vi "AWSEXE.vi"(8 "error in (no error)":errorcluster, 11 "DUT":string) -> (0 "error in (out)":errorcluster, 2 "Result":string)   [LabVIEW 2024, in "AWSEXE.lvlib"]
doc: "This template is for the Queued Message Handler design pattern.\n\nThe Event Handling Loop generates messages based on user interface actions.\n\nThe Message Handling Loop processes messages generated by the Event Handling Loop, or by other messages. The messages are string values, so new messages can be added easily to the Message Cases case structure in the Message Handling Loop. Each message cluster can also provide an optional value for Message Data, which is a variant that can be converted to whatever message-specific data is required."
uses:
  AWSEXE.lvlib
  support/Neoway_ctrl.ctl
  controls/Neoway UI Data.ctl
  PrivateControls/FGV_Queue_Control.ctl
  <vilib>/Utility/error.llb/Error Cluster From Error Code.vi
  <vilib>/ErrorRing/Error Ring.xnode
  support/Message Queue/Neoway Message Queue.lvlib
  support/User Event - Stop/72-13360 User Event - Stop.lvlib
  Launcher/Launcher_DTU.lvlib
panel:
  in  "Neoway Flashing":T1
  in  "Config":string
  in  "Read_Res":bool
  in  "Read_Current":bool
  in  "Read_File":bool
  in  "Flash":bool
  out "queue name 2":string
  out "queue name":string
  out "Display <Replace Me>":string
  in  "Output":bool
  in  "Init_Neoway":bool
  in  "Exit":bool
  # "These controls have associated \"Value Changed\" events configured in the Event Structure on the diagram.\n\nReplace them (and reconfigure the Event Structure) with the controls you need for your application."
  # "This template is for the Queued Message Handler design pattern.\n\nSee the block diagram for more information on how to use this template."
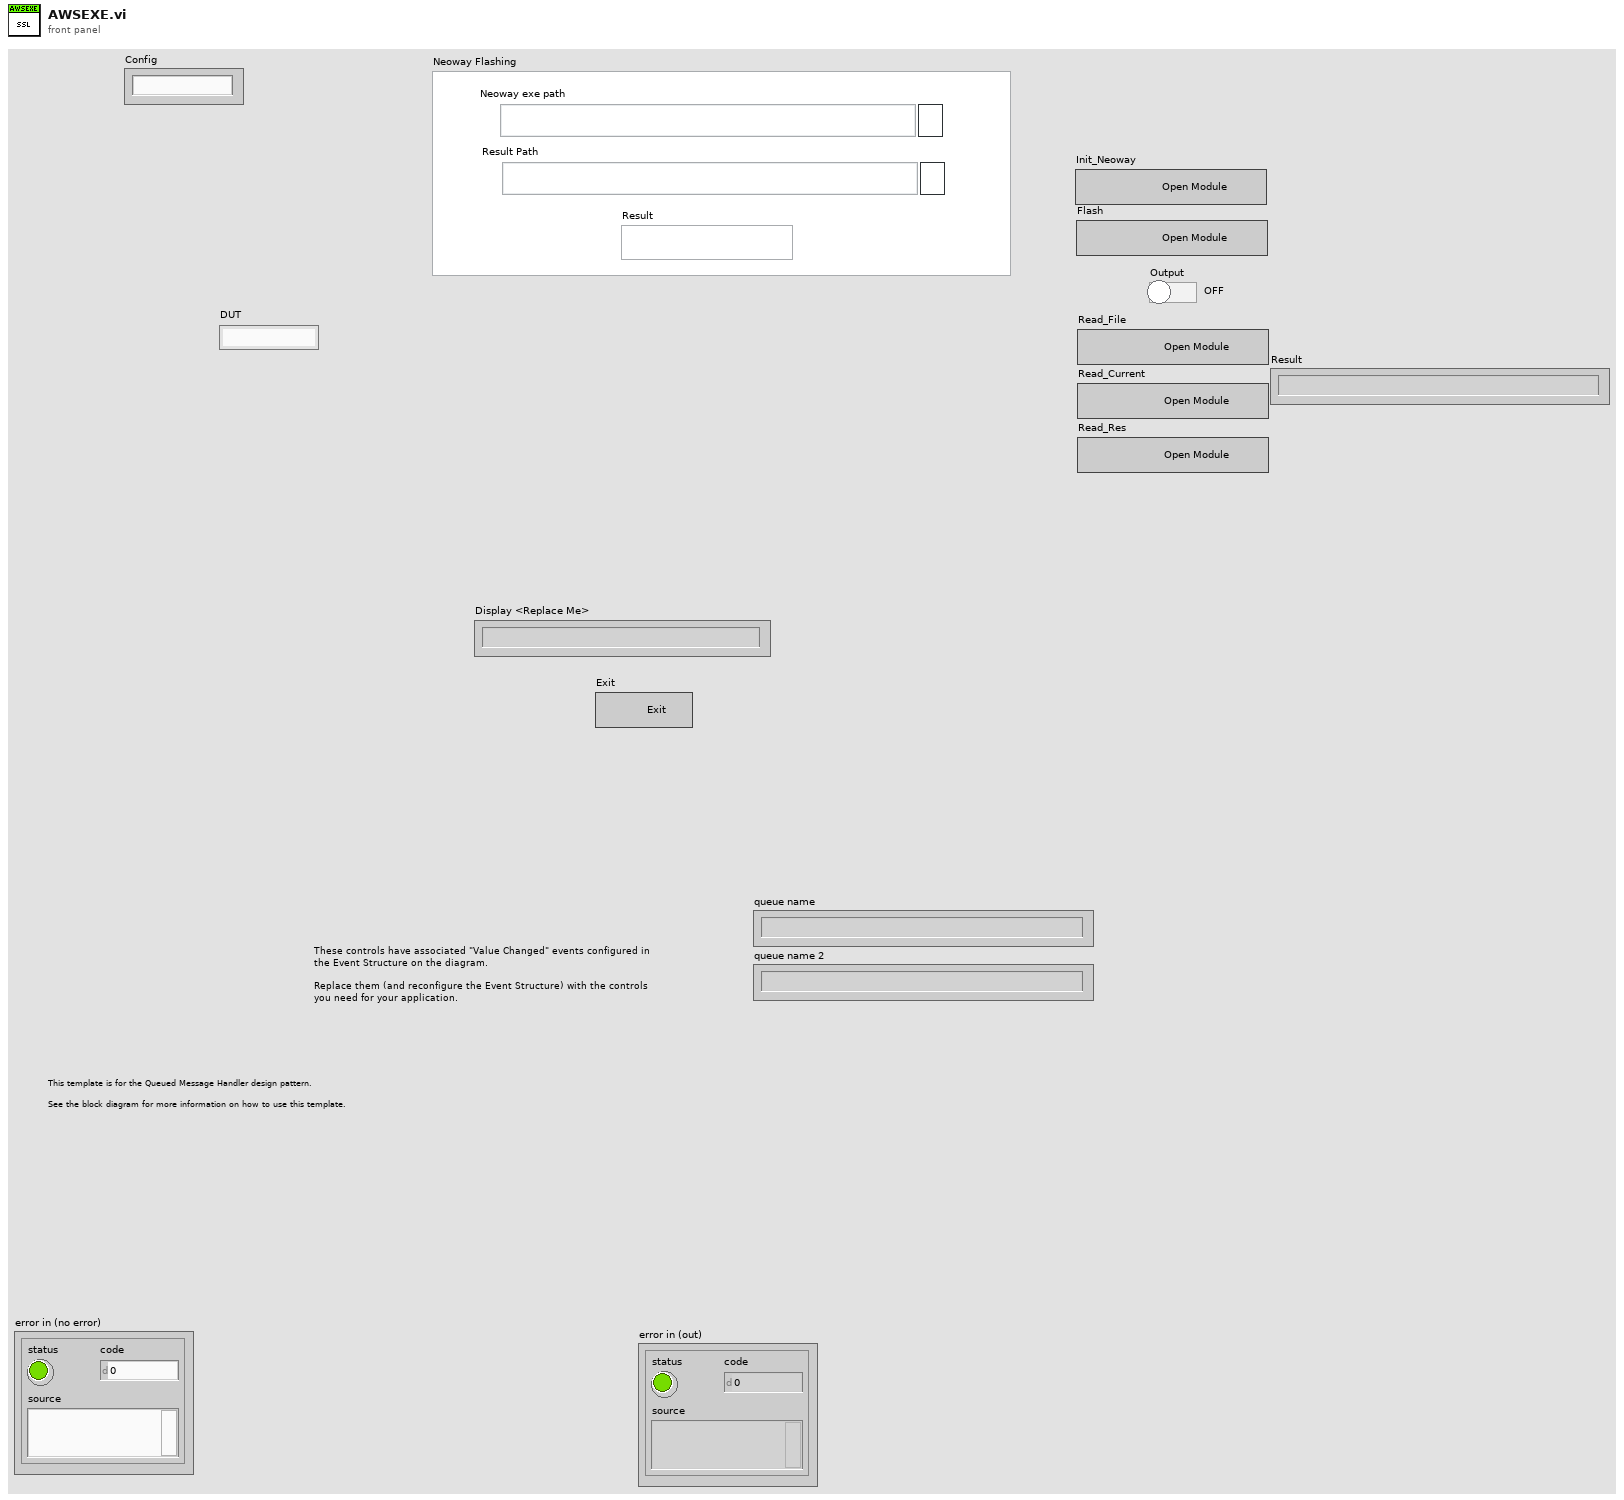
[diagram p1: front panel]
types:
  T1 = typedef "AWSEXE.lvlib/Neoway_ctrl.ctl" = cluster{"Neoway exe path":path, "Result Path":path, "Result":string}
  T2 = typedef "AWSEXE.lvlib/Neoway UI Data.ctl" = cluster{"DUT":string, "Neoway_Q":refnum<queue>, "notifier out":refnum<notifier>, "Config":string, "Neoway Flashing":T1, "Bat file path":path, "Exe path":string, "Flash path":string, "Result":string, "Timer":u32}
  T3 = typedef "AWSEXE.lvlib/FGV_Queue_Control.ctl" = enum16{"Release", "Get", "Set"}
  T4 = typedef "AWSEXE.lvlib/Neoway Message Queue.lvlib/All Message Queues.ctl" = cluster{"UI":refnum<queue>, "QSM":refnum<queue>}
  T5 = cluster{"Message":string, "Message Data":variant}
  T6 = enum16{"Read", "Write", "All_sections", "All_values", "Remove key&section"}
  T7 = enum16{"open", "replace", "create", "open or create", "replace or create", "replace or create with confirmation"}
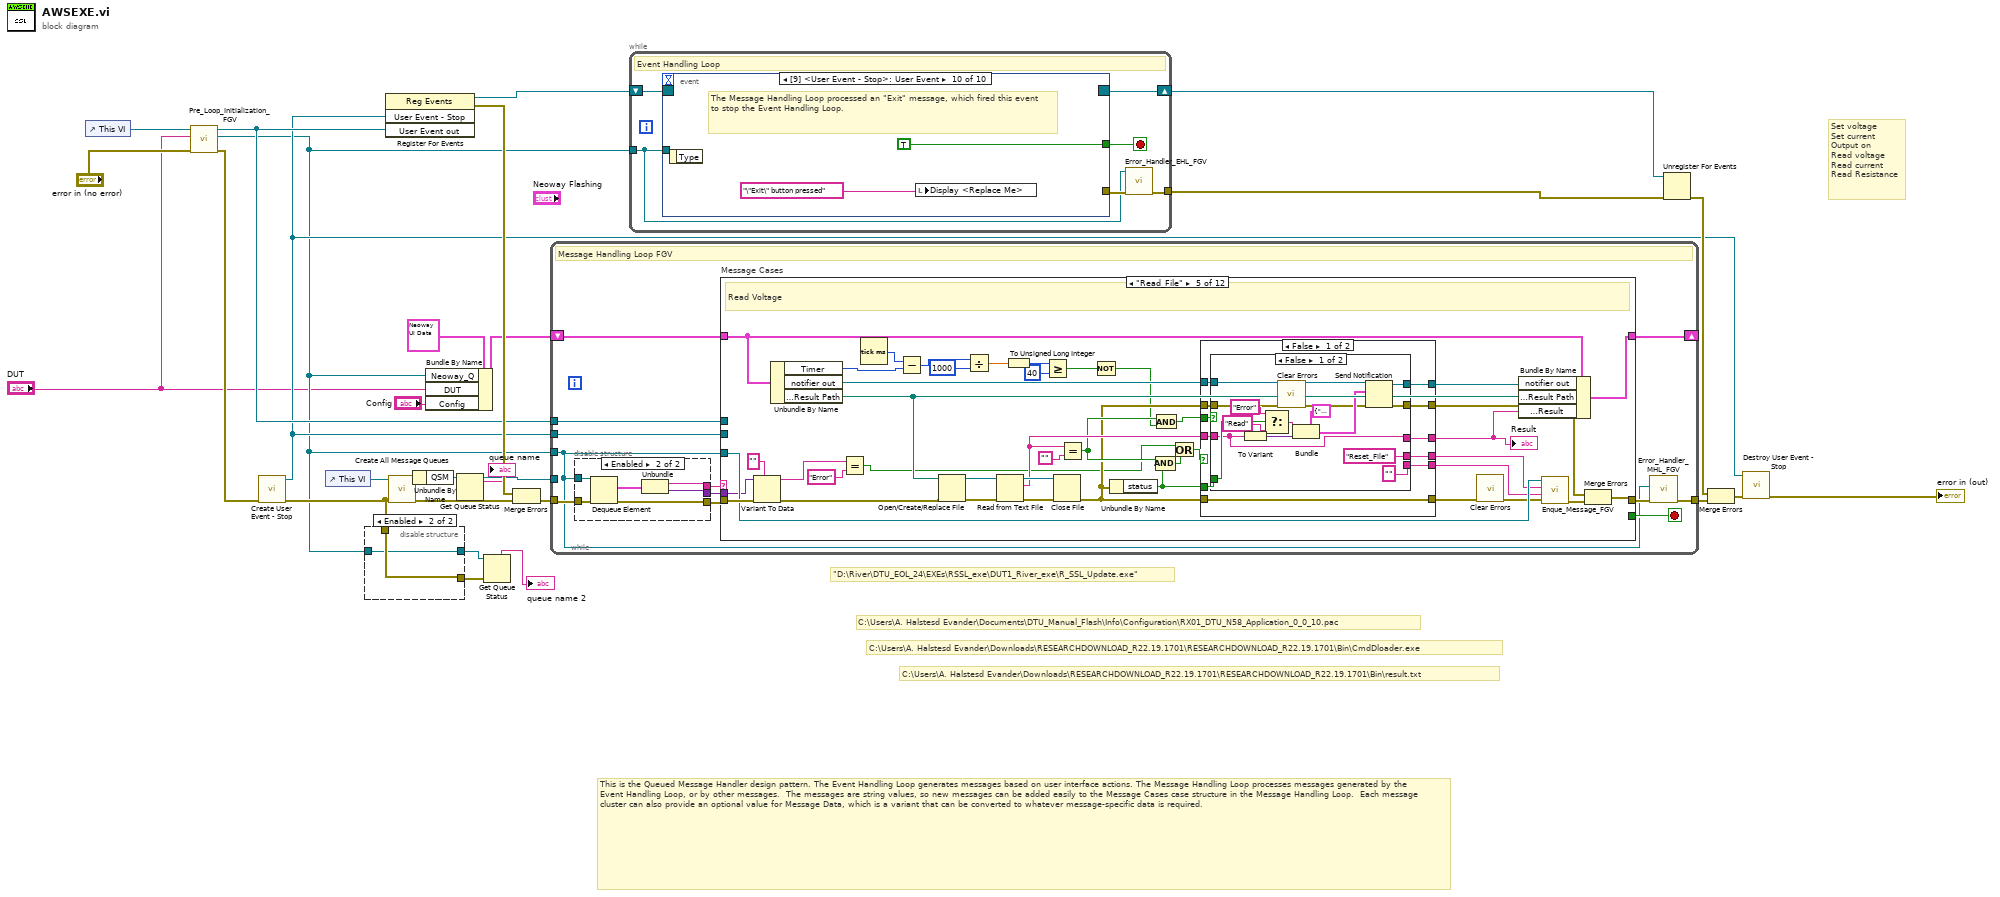
[diagram p0: block diagram]
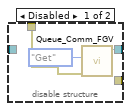
[diagram p2: hidden frame]
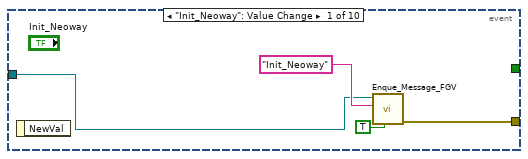
[diagram p3: hidden frame]
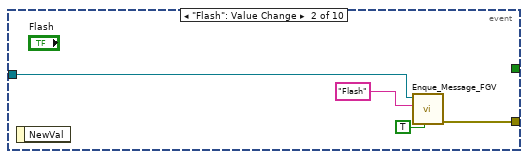
[diagram p4: hidden frame]
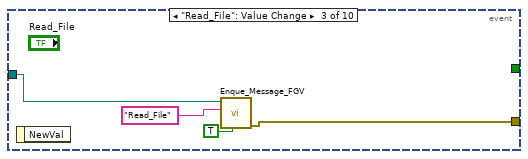
[diagram p5: hidden frame]
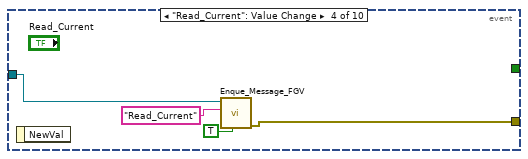
[diagram p6: hidden frame]
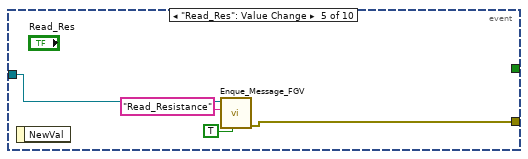
[diagram p7: hidden frame]
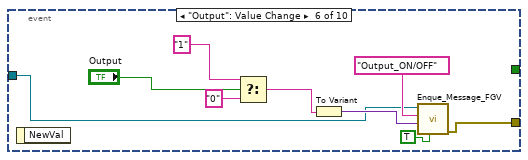
[diagram p8: hidden frame]
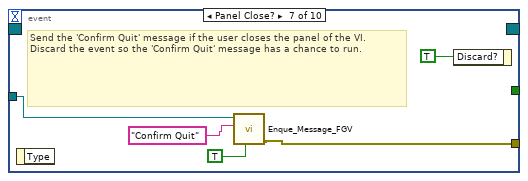
[diagram p9: hidden frame]
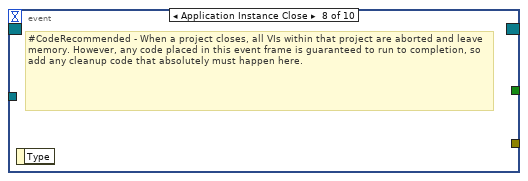
[diagram p10: hidden frame]
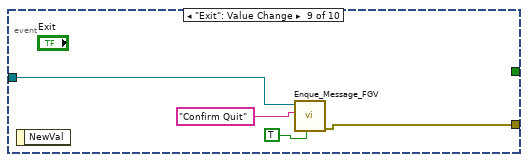
[diagram p11: hidden frame]
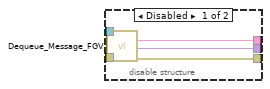
[diagram p12: hidden frame]
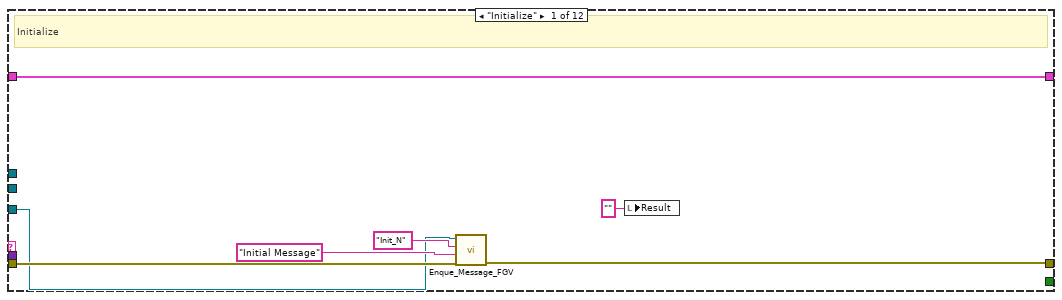
[diagram p13: hidden frame]
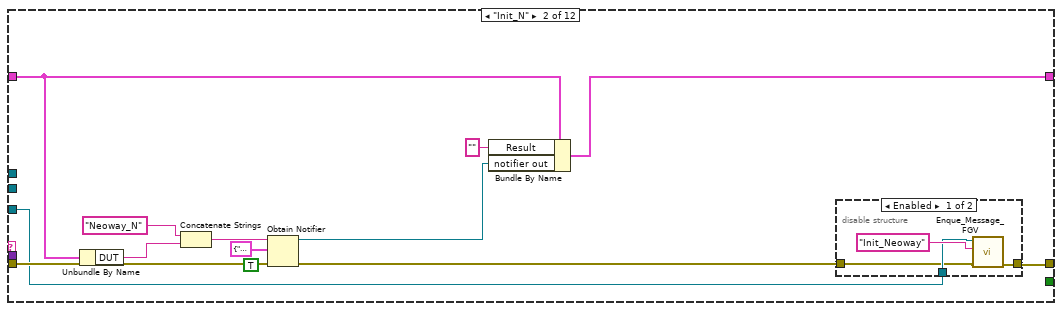
[diagram p14: hidden frame]
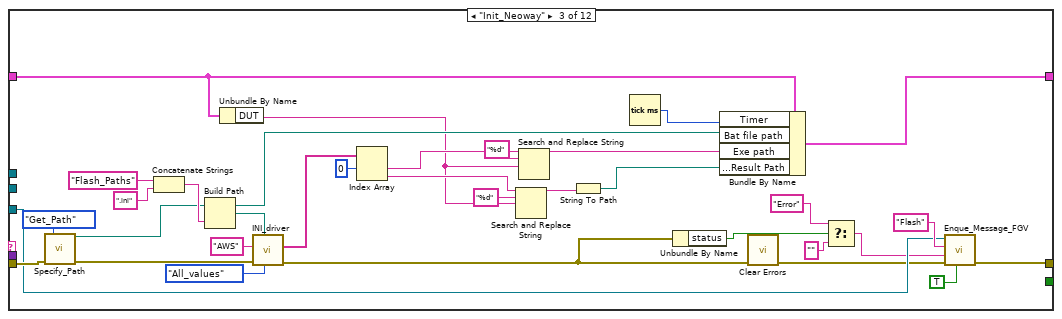
[diagram p16: hidden frame]
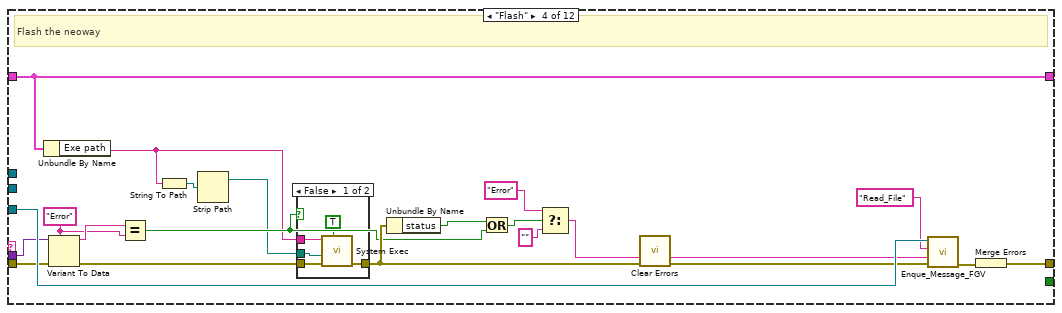
[diagram p17: hidden frame]
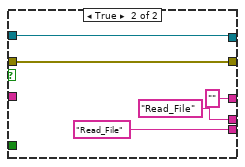
[diagram p19: hidden frame]
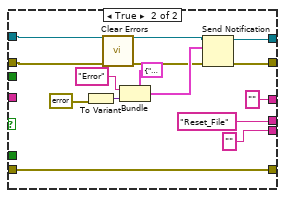
[diagram p20: hidden frame]
diagram:
  # "\"D:\\River\\DTU_EOL_24\\EXEs\\RSSL_exe\\DUT1_River_exe\\R_SSL_Update.exe\""
  # "C:\\Users\\A. Halstesd Evander\\Downloads\\RESEARCHDOWNLOAD_R22.19.1701\\RESEARCHDOWNLOAD_R22.19.1701\\Bin\\result.txt"
  # "C:\\Users\\A. Halstesd Evander\\Downloads\\RESEARCHDOWNLOAD_R22.19.1701\\RESEARCHDOWNLOAD_R22.19.1701\\Bin\\CmdDloader.exe"
  # "C:\\Users\\A. Halstesd Evander\\Documents\\DTU_Manual_Flash\\Info\\Configuration\\RX01_DTU_N58_Application_0_0_10.pac"
  # "Set voltage\nSet current\nOutput on\nRead voltage \nRead current\nRead Resistance"
  # "This is the Queued Message Handler design pattern. The Event Handling Loop generates messages based on user interface actions. The Message Handling Loop processes messages generated by the Event Handling Loop, or by other messages.  The messages are string values, so new messages can be added easily to the Message Cases case structure in the Message Handling Loop.  Each message cluster can also provide an optional value for Message Data, which is a variant that can be converted to whatever message-specific data is required."
  n1 = control-ref of="This VI"() -> (w17:refnum<vi>)
  n2 = call "Pre_Loop_Initialization_FGV.vi"("error in (no error)"="error in (no error)", "DUT"="DUT", "VI in"=w17) -> ("error out"=w15:errorcluster, "queue out"=w3:refnum<queue>, "User Event out"=w7:refnum<user-event>)  [unwired: 6 in]
  n3 = call "Create User Event - Stop.vi"("error in (no error)"=w15) -> ("error out"=w10:errorcluster, "User Event - Stop"=w6:refnum<user-event>)  [unwired: 9 in]
  n4 = control-ref of="This VI"() -> (w13:refnum<vi>)
  n5 = disable-structure shown="Enabled" {
    disable-tunnel: w10 -> [w32 w34]
    disable-tunnel: [w30 w33] -> w9
    disable-tunnel: [_ w34] -> w5
    disable-tunnel: w3 -> [_ w33]
    frame Disabled {
      n6 = call "Queue_Comm_FGV.vi"("error in (no error)"=w32, "Enum"=FGV_Queue_Control."Get") -> ("queue Out"=w30:refnum<queue>)  [unwired: 8 in, 1 out]
    }
    frame Enabled {
    }
  }
  n7 = register-events(w6, w7) -> (reference out=w20:refnum<event-registration>, error out=w18:errorcluster)  [unwired: 2 in]
  n8 = call "Create All Message Queues.vi"("error in (no error)"=w10, "This VI"=w13) -> ("error out"=w29:errorcluster, "Message Queues out"=w28:T4)  [unwired: 8 in]
  n9 = Unbundle By Name(w28) -> ("QSM"=w26:refnum<queue>)
  n10 = Bundle By Name(cluster=T2 {"DUT"="", "Neoway_Q"=refnum, "notifier out"=refnum, "Config"="", "Neoway Flashing"={"Neoway exe path"=path "", "Result Path"=path "", "Result"=""}, "Bat file path"=path "", "Exe path"="", "Flash path"="", "Result"="", "Timer"=0} ("Data Cluster"), "Neoway_Q"=w3, "DUT"="DUT", "Config"="Config") -> (w4:T2)
  n11 = Get Queue Status(queue=w26) -> (queue out=w12:refnum<queue>, queue name=→"queue name":string)  [unwired: 2 in, 6 out]
  n12 = Get Queue Status(queue=w9, error in (no error)=w5) -> (queue name=→"queue name 2":string)  [unwired: 1 in, 7 out]
  n13 = Merge Errors(w18, w29) -> (w19:errorcluster)
  n14 = while {
    tunnel: w12 -> [_]
    shift-right: [w45] -> _
    shift-left: w4 -> [w46]
    tunnel: w7 -> [w43]
    tunnel: w19 -> [w42]
    tunnel: [w37] -> w27
    tunnel: w6 -> [w36]
    tunnel: w3 -> [w35]
    stop <- w44 stop-if-true
    # "Message Handling Loop FGV"
    n15 = disable-structure shown="Enabled" {
      disable-tunnel: w42 -> [w50 w56]
      disable-tunnel: [w49 w54] -> w41
      disable-tunnel: [w48 w51] -> w40
      disable-tunnel: [w47 w52] -> w39
      disable-tunnel: w35 -> [_ w55]
      frame Disabled {
        n16 = call "Dequeue_Message_FGV.vi"("error in (no error)"=w50) -> ("error out"=w49:errorcluster, "Message Data"=w48:variant, "Message"=w47:string)  [unwired: 8 in]
      }
      frame Enabled {
        n17 = Dequeue Element(queue=w55, error in (no error)=w56) -> (element=w53:T5, error out=w54:errorcluster)  [unwired: 1 in, 2 out]
        n18 = Unbundle(w53) -> ("Message"=w52:string, "Message Data"=w51:variant)
      }
    }
    n19 = case "Message Cases" shown="\"Read_File\"" w39 {
      selector: w39 -> [_ _ _ _ _ _ _ _ _ _ _ w293]
      tunnel: w41 -> [w59 w76 w114 w132 w183 w243 w253 w262 w271 w276 w284 _]
      tunnel: [w62 w65 w90 w135 w178 w230 w245 w260 w273 w274 w277 w294] -> w38
      tunnel: w46 -> [w63 w74 w99 w131 w181 w242 w254 w261 w268 w275 w279 w295]
      tunnel: [w63 w69 w104 w131 w180 w242 w254 w261 w268 w275 w279 w295] -> w45
      tunnel: [_ _ _ _ _ _ _ _ _ _ TRUE _] -> w44
      tunnel: w40 -> [_ _ _ w122 w177 _ w252 _ _ _ w286 _]
      tunnel: w43 -> [_ _ _ _ _ _ _ _ _ _ w287 _]
      tunnel: w36 -> [_ _ _ _ _ _ _ _ _ _ w282 _]
      tunnel: w35 -> [w58 w67 w89 w133 w179 w229 w244 w255 w266 _ w278 _]
      frame "Initialize" {
        # "Initialize"
        n20 = call "Enque_Message_FGV.vi"("error in (no error)"=w59, "Message Data"="Initial Message" ("Initial Message"), "Message"="Init_N", "queue in"=w58) -> ("error out"=w62:errorcluster)  [unwired: 7 in]
        n21 = local write "Result"("" ("Result")) -> ()
      }
      frame "Init_N" {
        n22 = Unbundle By Name(w74) -> ("DUT"=w73:string)
        n23 = Concatenate Strings("Neoway_N", w73) -> (w72:string)
        n24 = Obtain Notifier(name (unnamed)=w72, notification data type=T5 {"Message"="", "Message Data"=variant} ("notification"), create if not found? (T)=TRUE, error in (no error)=w76) -> (notifier out=w68:refnum<notifier>, error out=w66:errorcluster)  [unwired: 1 out]
        n25 = Bundle By Name(cluster=w74, "Result"="", "notifier out"=w68) -> (w69:T2)
        n26 = disable-structure shown="Enabled" {
          disable-tunnel: w67 -> [w79 _]
          disable-tunnel: w66 -> [w78 w81]
          disable-tunnel: [w77 w81] -> w65
          frame Enabled {
            n27 = call "Enque_Message_FGV.vi"("error in (no error)"=w78, "Message"="Init_Neoway", "queue in"=w79) -> ("error out"=w77:errorcluster)  [unwired: 8 in]
          }
          frame Disabled {
          }
        }
      }
      frame "Init_Neoway" {
        n28 = call "Specify_Path.vi"("Path_Enum"=enum16{"Find_Path", "Get_Path"}."Get_Path", "error in (no error)"=w114) -> ("Configurations"=w102:path, "error out"=w109:errorcluster)  [unwired: 6 in, 6 out]
        n29 = Concatenate Strings("Flash_Paths" ("string"), ".ini" ("string")) -> (w111:string)
        n30 = Build Path(base path=w102, name or relative path=w111) -> (appended path=w110:path)
        n31 = Unbundle By Name(w99) -> ("DUT"=w95:string)
        n32 = call "INI_driver.vi"("Enum"=T6."All_values", "instrument file path"=w110, "error in (no error)"=w109, "Section"="AWS") -> ("error out"=w85:errorcluster, "Values out"=w107:string[])  [unwired: 4 in, 2 out]
        n33 = Index Array(array=w107, index #1=0 ("index")) -> (element #1=w101:string, element #2=w96:string)  [unwired: 1 in]
        n34 = Search and Replace String(input string=w96, search string="%d", replace string=w95) -> (result string=w94:string)  [unwired: 5 in, 3 out]
        n35 = Search and Replace String(input string=w101, search string="%d", replace string=w95) -> (result string=w98:string)  [unwired: 5 in, 3 out]
        n36 = String To Path(string=w94) -> (path=w93:path)
        n37 = Tick Count (ms)() -> (millisecond timer value=w82:u32)
        n38 = Unbundle By Name(w85) -> ("status"=w87:bool)
        n39 = Bundle By Name(cluster=w99, "Timer"=w82, "Bat file path"=w102, "Exe path"=w98, "Neoway Flashing.Result Path"=w93) -> (w104:T2)
        n40 = call <vilib>:"Clear Errors.vi"("error in (no error)"=w85) -> ("error out"=w83:errorcluster)  [unwired: 5 in, 1 out]
        n41 = Select(t="Error" ("\"Do Something\" button pressed"), s=w87, f="" ("\"Do Something\" button pressed")) -> (s? t:f=w84:string)
        n42 = call "Enque_Message_FGV.vi"("Priority"=TRUE ("Priority Message? (F)"), "error in (no error)"=w83, "Message Data"=w84, "Message"="Flash", "queue in"=w89) -> ("error out"=w90:errorcluster)  [unwired: 6 in]
      }
      frame "Flash" {
        w119 = "Error" ("Message")
        # "Flash the neoway"
        n43 = Unbundle By Name(w131) -> ("Exe path"=w117:string)
        n44 = Variant To Data(error in=w132, type=w119, Variant=w122) -> (data=w120:string, error out=w123:errorcluster)
        n45 = Equal?(x=w120, y=w119) -> (x = y?=w118:bool)
        n46 = String To Path(string=w117) -> (path=w116:path)
        n47 = Strip Path(path=w116) -> (stripped path=w115:path)  [unwired: 1 out]
        n48 = case shown="False" w118 {
          tunnel: w117 -> [w140 _]
          tunnel: [w139 w141] -> w130
          tunnel: w123 -> [w138 w141]
          tunnel: w115 -> [w136 _]
          frame False {
            n49 = call <vilib>:"System Exec.vi"("wait until completion? (T)"=TRUE, "error in (no error)"=w138, "working directory"=w136, "command line"=w140) -> ("error out"=w139:errorcluster)  [unwired: 4 in, 3 out]
          }
          frame True {
          }
        }
        n50 = Unbundle By Name(w130) -> ("status"=w127:bool)
        n51 = Or(x=w127, y=w118) -> (x .or. y?=w121:bool)
        n52 = Select(t="Error" ("\"Do Something\" button pressed"), s=w121, f="" ("\"Do Something\" button pressed")) -> (s? t:f=w125:string)
        n53 = call <vilib>:"Clear Errors.vi"("error in (no error)"=w130) -> ("error out"=w124:errorcluster)  [unwired: 5 in, 1 out]
        n54 = call "Enque_Message_FGV.vi"("error in (no error)"=w124, "Message Data"=w125, "Message"="Read_File", "queue in"=w133) -> ("error out"=w134:errorcluster)  [unwired: 7 in]
        n55 = Merge Errors(w134) -> (w135:errorcluster)
      }
      frame "Read_File" {
        # "Read Voltage"
        n56 = Variant To Data(error in=w183, type="", Variant=w177) -> (data=w174:string, error out=w173:errorcluster)
        n57 = Unbundle By Name(w181) -> ("Timer"=w151:u32, "notifier out"=w164:refnum<notifier>, "Neoway Flashing.Result Path"=w167:path)
        n58 = Equal?(x=w174, y="Error" ("\"Do Something\" button pressed")) -> (x = y?=w155:bool)
        n59 = Tick Count (ms)() -> (millisecond timer value=w152:u32)
        n60 = Subtract(x=w152, y=w151) -> (x-y=w150:u32)
        n61 = Open/Create/Replace File(file path (use dialog)=w167, error in=w173) -> (refnum out=w170:refnum<file>, error out=w172:errorcluster)  [unwired: 4 in, 1 out]
        n62 = Divide(x=w150, y=u32 1000) -> (x/y=w148:dbl)
        n63 = Read from Text File(file (use dialog)=w170, error in=w172) -> (refnum out=w168:refnum<file>, text=w162:string, error out=w171:errorcluster)  [unwired: 2 in, 1 out]
        n64 = To Unsigned Long Integer(number=w148) -> (unsigned 32bit integer=w147:u32)
        n65 = Greater Or Equal?(x=w147, y=u32 40) -> (x >= y?=w144:bool)
        n66 = Close File(refnum=w168, error in=w171) -> (error out=w157:errorcluster)  [unwired: 1 out]
        n67 = Equal?(x=w162, y="") -> (x = y?=w160:bool)
        n68 = Not(x=w144) -> (.not. x?=w142:bool)
        n69 = Unbundle By Name(w157) -> ("status"=w161:bool)
        n70 = And(x=w160, y=w142) -> (x .and. y?=w145:bool)
        n71 = Compound Arithmetic op=AND(w160, w161) -> (w154:bool)
        n72 = Or(x=w155, y=w154) -> (x .or. y?=w153:bool)
        n73 = case shown="False" w153 {
          tunnel: w157 -> [w194 w220]
          tunnel: [w193 w221] -> w165
          tunnel: w164 -> [w192 w223]
          tunnel: [w191 w222] -> w163
          tunnel: w162 -> [w190 _]
          tunnel: w161 -> [w189 _]
          tunnel: w145 -> [w188 _]
          tunnel: [w187 "Reset_File" ("Message")] -> w159
          tunnel: [w186 "" ("\"Do Something\" button pressed")] -> w158
          tunnel: w157 -> [w185 w228]
          tunnel: [w185 w228] -> w156
          tunnel: [w184 ""] -> w143
          frame False {
            n74 = case shown="False" w188 {
              tunnel: w194 -> [w203 w214]
              tunnel: [w201 w214] -> w193
              tunnel: w192 -> [w200 w213]
              tunnel: [w199 w213] -> w191
              tunnel: w190 -> [w195 _]
              tunnel: w189 -> [w198 _]
              tunnel: ["Reset_File" ("Message") "Read_File" ("Message")] -> w187
              tunnel: ["" ("\"Do Something\" button pressed") "Read_File" ("\"Do Something\" button pressed")] -> w186
              tunnel: [w195 ""] -> w184
              frame False {
                n75 = To Variant(anything=w195) -> (Variant=w208:variant)
                n76 = Select(t="Error" ("f"), s=w198, f="Read" ("Message")) -> (s? t:f=w209:string)
                n77 = call <vilib>:"Clear Errors.vi"("error in (no error)"=w203) -> ("error out"=w202:errorcluster)  [unwired: 5 in, 1 out]
                n78 = Bundle(cluster=T5 {"Message"="", "Message Data"=variant} ("notification"), "Message"=w209, "Message Data"=w208) -> (w207:T5)
                n79 = Send Notification(notification=w207, notifier=w200, error in (no error)=w202) -> (notifier out=w199:refnum<notifier>, error out=w201:errorcluster)
              }
              frame True {
              }
            }
          }
          frame True {
            n80 = To Variant(anything=errorcluster {"status"=TRUE, "code"=0, "source"="Error at N58 Flashing"} ("error constant")) -> (Variant=w227:variant)
            n81 = call <vilib>:"Clear Errors.vi"("error in (no error)"=w220) -> ("error out"=w224:errorcluster)  [unwired: 5 in, 1 out]
            n82 = Bundle(cluster=T5 {"Message"="", "Message Data"=variant} ("notification"), "Message"="Error" ("f"), "Message Data"=w227) -> (w226:T5)
            n83 = Send Notification(notification=w226, notifier=w223, error in (no error)=w224) -> (notifier out=w222:refnum<notifier>, error out=w221:errorcluster)
          }
        }
        "Result" <- w143
        n84 = call <vilib>:"Clear Errors.vi"("error in (no error)"=w156) -> ("error out"=w166:errorcluster)  [unwired: 5 in, 1 out]
        n85 = Bundle By Name(cluster=w181, "notifier out"=w163, "Neoway Flashing.Result Path"=w167, "Neoway Flashing.Result"=w143) -> (w180:T2)
        n86 = call "Enque_Message_FGV.vi"("error in (no error)"=w166, "Message Data"=w158, "Message"=w159, "queue in"=w179) -> ("error out"=w182:errorcluster)  [unwired: 7 in]
        n87 = Merge Errors(w165, w182) -> (w178:errorcluster)
      }
      frame "Reset_File" {
        n88 = Unbundle By Name(w242) -> ("Neoway Flashing.Result Path"=w240:path)  [unwired: 1 out]
        n89 = Open/Create/Replace File(file path (use dialog)=w240, error in=w243, operation (0:open)=T7."replace") -> (refnum out=w237:refnum<file>, error out=w241:errorcluster)  [unwired: 3 in, 1 out]
        n90 = Read from Text File(file (use dialog)=w237, error in=w241) -> (refnum out=w234:refnum<file>, text=w235:string, error out=w238:errorcluster)  [unwired: 2 in, 1 out]
        n91 = Equal?(x=w235, y="") -> ()  [unwired: 1 out]
        n92 = Close File(refnum=w234, error in=w238) -> (error out=w231:errorcluster)  [unwired: 1 out]
        n93 = call "Enque_Message_FGV.vi"("error in (no error)"=w231, "Message Data"="Resetted Flash file" ("\"Do Something\" button pressed"), "Message"="Update Display", "queue in"=w229) -> ("error out"=w230:errorcluster)  [unwired: 7 in]
      }
      frame "Update Display" {
        # "#CodeRecommended - If you wish to decouple the Message Handling Loop from your user interface, consider creating User Events (like the \"Stop\" event in this VI) to message the Event Handling Loop whenever the user interface needs updating."
        # "Update Display - Convert the message data to a string to display in the Data Display indicator."
        n94 = Variant To Data(error in=w253, type="", Variant=w252) -> (data=→"Display <Replace Me>":string, error out=w250:errorcluster)
        n95 = call <vilib>:"Clear Errors.vi"("error in (no error)"=w250) -> ("error out"=w248:errorcluster)  [unwired: 5 in, 1 out]
        n96 = Merge Errors(w248) -> (w246:errorcluster)
        n97 = call "Enque_Message_FGV.vi"("error in (no error)"=w246, "Message"="Confirm Quit", "queue in"=w244) -> ("error out"=w245:errorcluster)  [unwired: 8 in]
      }
      frame "Error" {
        # "Error - Display an error dialog. This message is sent by the \"Error Handler\" VIs at the end of other loops in this application."
        n98 = call <vilib>:"Clear Errors.vi"("error in (no error)"=w262) -> ("error out"=w257:errorcluster)  [unwired: 5 in, 1 out]
        n99 = call "Enque_Message_FGV.vi"("Priority"=TRUE ("Priority Message? (F)"), "error in (no error)"=w257, "Message"="Confirm Quit", "queue in"=w255) -> ("error out"=w256:errorcluster)  [unwired: 7 in]
        n100 = Merge Errors(w256) -> (w260:errorcluster)
      }
      frame "Confirm Quit" {
        # "Confirm Quit - Message that can confirm whether or not the user wants to exit the application."
        n101 = Unbundle By Name(w268) -> ("notifier out"=w264:refnum<notifier>)
        n102 = Release Notifier(notifier=w264, force destroy? (F)=TRUE, error in (no error)=w271) -> (error out=w265:errorcluster)  [unwired: 2 out]
        n103 = call <vilib>:"Clear Errors.vi"("error in (no error)"=w265) -> ("error out"=w267:errorcluster)  [unwired: 5 in, 1 out]
        n104 = call "Enque_Message_FGV.vi"("Priority"=TRUE ("Priority Message? (F)"), "error in (no error)"=w267, "Message"="Exit", "queue in"=w266) -> ("error out"=w272:errorcluster)  [unwired: 7 in]
        n105 = Merge Errors(w272) -> (w273:errorcluster)
      }
      frame "---Copy This Frame---" {
        # "Duplicate this frame when creating new messages.  Change this comment in the duplicated frame to describe this message."
        n106 = Merge Errors(w276) -> (w274:errorcluster)
      }
      frame "Exit" {
        # "Stop the VI"
        # "Release the message queue reference"
        # "Exit - Exit the application."
        n107 = disable-structure shown="Enabled" {
          disable-tunnel: w286 -> [w290 _]
          frame Disabled {
            n108 = Variant To Data(type=errorcluster {"status"=FALSE, "code"=0, "source"=""} ("error constant"), Variant=w290) -> (data=w291:errorcluster)  [unwired: 1 in, 1 out]
            n109 = call <vilib>:"Simple Error Handler.vi"("error in (no error)"=w291) -> ()  [unwired: 4 in, 5 out]
          }
          frame Enabled {
          }
        }
        n110 = call "Queue_Comm_FGV.vi"("error in (no error)"=w284, "Enum"=FGV_Queue_Control."Release", "queue in"=w278) -> ("error Out"=w283:errorcluster)  [unwired: 7 in, 1 out]
        n111 = call "Fire User Event - Stop.vi"("User Event - Stop"=w282) -> ("error out"=w280:errorcluster)  [unwired: 10 in]
        n112 = call "Fire User Event - Stop.vi"("User Event - Stop"=w287) -> ("error out"=w281:errorcluster)  [unwired: 10 in]
        n113 = Merge Errors(w281, w280, w283) -> (w288:errorcluster)
        n114 = call <vilib>:"Clear Errors.vi"("error in (no error)"=w288) -> ("error out"=w277:errorcluster)  [unwired: 5 in, 1 out]
      }
      frame Default {
        # "'Default' case only runs if there is a message that isn't defined in any of the other cases.  Output a programming error."
        n115 = xnode "Error Ring"("parameter 0"=w293) -> ("error out"=w294:errorcluster)
      }
    }
    n116 = call "Error_Handler_MHL_FGV.vi"("error in (no error)"=w38, "queue in"=w35) -> ("error Out"=w37:errorcluster)  [unwired: 9 in]
  }
  n117 = while {
    shift-right: [w307] -> w23
    shift-left: w20 -> [w308]
    tunnel: [w304] -> w21
    tunnel: w3 -> [w303]
    stop <- w306 stop-if-true
    # "Event Handling Loop"
    n118 = event shown="[9] <User Event - Stop>: User Event" {
      selector: w308 -> [_ _ _ _ _ _ _ _ _ _]
      dyn-events: [_ _ _ _ _ _ _ _ _ _] -> w307
      timeout: _ -> [_ _ _ _ _ _ _ _ _ _]
      tunnel: [_ _ _ _ _ _ _ _ _ TRUE ("Discard?")] -> w306
      tunnel: [w311 w315 w319 w323 w327 w335 w341 _ w346 _] -> w305
      tunnel: w303 -> [w309 w313 w317 w321 w325 w329 w338 _ w343 _]
      event "Init_Neoway": Value Change {
        n119 = event-data() -> ()  [unwired: 1 in, 1 out]
        n120 = call "Enque_Message_FGV.vi"("Priority"=TRUE ("Priority Message? (F)"), "Message"="Init_Neoway", "queue in"=w309) -> ("error out"=w311:errorcluster)  [unwired: 8 in]
      }
      event "Flash": Value Change {
        n121 = event-data() -> ()  [unwired: 1 in, 1 out]
        n122 = call "Enque_Message_FGV.vi"("Priority"=TRUE ("Priority Message? (F)"), "Message"="Flash", "queue in"=w313) -> ("error out"=w315:errorcluster)  [unwired: 8 in]
      }
      event "Read_File": Value Change {
        n123 = event-data() -> ()  [unwired: 1 in, 1 out]
        n124 = call "Enque_Message_FGV.vi"("Priority"=TRUE ("Priority Message? (F)"), "Message"="Read_File", "queue in"=w317) -> ("error out"=w319:errorcluster)  [unwired: 8 in]
      }
      event "Read_Current": Value Change {
        n125 = event-data() -> ()  [unwired: 1 in, 1 out]
        n126 = call "Enque_Message_FGV.vi"("Priority"=TRUE ("Priority Message? (F)"), "Message"="Read_Current", "queue in"=w321) -> ("error out"=w323:errorcluster)  [unwired: 8 in]
      }
      event "Read_Res": Value Change {
        n127 = event-data() -> ()  [unwired: 1 in, 1 out]
        n128 = call "Enque_Message_FGV.vi"("Priority"=TRUE ("Priority Message? (F)"), "Message"="Read_Resistance", "queue in"=w325) -> ("error out"=w327:errorcluster)  [unwired: 8 in]
      }
      event "Output": Value Change {
        n129 = event-data() -> ()  [unwired: 1 in, 1 out]
        n130 = Select(t="1", s="Output", f="0") -> (s? t:f=w331:string)
        n131 = To Variant(anything=w331) -> (Variant=w330:variant)
        n132 = call "Enque_Message_FGV.vi"("Priority"=TRUE ("Priority Message? (F)"), "Message Data"=w330, "Message"="Output_ON/OFF", "queue in"=w329) -> ("error out"=w335:errorcluster)  [unwired: 7 in]
      }
      event Panel Close? {
        # "Send the 'Confirm Quit' message if the user closes the panel of the VI. Discard the event so the 'Confirm Quit' message has a chance to run."
        n133 = event-data() -> ()  [unwired: 1 in, 1 out]
        n134 = call "Enque_Message_FGV.vi"("Priority"=TRUE ("Priority Message? (F)"), "Message"="Confirm Quit", "queue in"=w338) -> ("error out"=w341:errorcluster)  [unwired: 8 in]
        n135 = event-data("Discard?"=TRUE) -> ()  [unwired: 1 in, 1 out]
      }
      event Application Instance Close {
        # "#CodeRecommended - When a project closes, all VIs within that project are aborted and leave memory. However, any code placed in this event frame is guaranteed to run to completion, so add any cleanup code that absolutely must happen here."
        n136 = event-data() -> ()  [unwired: 1 in, 1 out]
      }
      event "Exit": Value Change {
        n137 = event-data() -> ()  [unwired: 1 in, 1 out]
        n138 = call "Enque_Message_FGV.vi"("Priority"=TRUE ("Priority Message? (F)"), "Message"="Confirm Quit", "queue in"=w343) -> ("error out"=w346:errorcluster)  [unwired: 8 in]
      }
      event User Event {
        # "The Message Handling Loop processed an \"Exit\" message, which fired this event to stop the Event Handling Loop."
        n139 = event-data() -> ()  [unwired: 1 in, 1 out]
        n140 = local write "Display <Replace Me>"("\"Exit\" button pressed" ("VI Stopped")) -> ()
      }
    }
    n141 = call "Error_Handler_EHL_FGV.vi"("error in (no error)"=w305, "queue in"=w303) -> ("error Out"=w304:errorcluster)  [unwired: 9 in]
  }
  n142 = Unregister For Events(event registration refnum=w23, error in=w21) -> (error out=w24:errorcluster)
  n143 = Merge Errors(w24, w27) -> (w25:errorcluster)
  n144 = call "Destroy User Event - Stop.vi"("error in (no error)"=w25, "User Event - Stop"=w6) -> ("error out"=→"error in (out)":errorcluster)  [unwired: 9 in]
